vi "Method 1 Ultrasonic.vi"   [LabVIEW 2012]
uses:
  <vilib>/NXT/Subs/MotorOutput.ctl
  <vilib>/NXT/Block Support/NXT_InputPort.ctl
types:
  T1 = typedef "NXT_InputPort.ctl" = u32
  T2 = typedef "MotorOutput.ctl" = u8
  T3 = typedef "LVHSConnector.ctl" = refnum<class "BrickReference.lvclass">
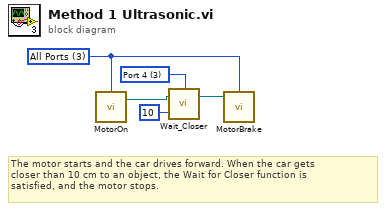
[diagram p0: block diagram]
diagram:
  w4 = T1 3 items=["Port 1", "Port 2", "Port 3", "Port 4"] ("Port (Port 4)")
  w5 = T2 3 items=["Port A", "Port B", "Port C", "All Ports"] ("Output Port")
  # "The motor starts and the car drives forward. When the car gets\ncloser than 10 cm to an object, the Wait for Closer function is\nsatisfied, and the motor stops."
  n1 = call <vilib>:"MotorOn.vi"("Output Port (All Ports)"=w5) -> ("NXT/EV3"=w3:T3)  [unwired: 3 in]
  n2 = call <vilib>:"Wait_Closer.vi"("Distance (40)"=i16 10, "NXT/EV3"=w3, "Port (Port 4)"=w4) -> ("NXT/EV3"=w2:T3)  [unwired: 1 in]
  n3 = call <vilib>:"MotorBrake.vi"("NXT/EV3"=w2, "Port (All Ports)"=w5) -> ()  [unwired: 2 in, 1 out]
